vi "Ctr sys net adapter port auto detect.vi"(11 "HW Config IN":T1={"Dev. PC"=FALSE, "Swap XY on stage"=FALSE, "No of AOD"=0, "MC Supported"=FALSE, "Axial MC"=FALSE, "Computer MAC address"="", "Externalise Triggers"=FALSE, "Trigger HW config"={"Available Device List"=0, "Device Address"=""}, "DAQmx Chan"={"Pockels AO"="", "Hard shutter AO"="", "PMT AOs"="", "Galvo AOs"="", "Power meter AI"=""}, "XYZ Stage Control Config"=enum."None", "XY stage available"=FALSE, "XY Comms Config Cluster"={"Name"="COM7", "Device Address"="", "Port "=0, "Baudrate"=0, "Comms Type"=enum."GPIB-IEEE488"}, "Y stage available"=FALSE, "Y Comms Config Cluster"={"Name"="", "Device Address"="", "Port "=0, "Baudrate"=0, "Comms Type"=enum."GPIB-IEEE488"}, "Z stage available"=FALSE, "Z Comms Config Cluster "={"Name"="", "Device Address"="", "Port "=0, "Baudrate"=0, "Comms Type"=enum."GPIB-IEEE488"}, "Encoder available"=FALSE, "Encoder"={"IP address"="224.0.1.103", "Port"=7000, "Wheel radius (cm)"=16.0, "Encoder Trigger"=""}, "VidRec available"=FALSE, "Cam VidRec"={"DO flag-Video record"="", "DO flag-Trial start"=""}, "Laser Power Control HW config"={"Laser Power Control"="", "Laser Power Modulation Control"=enum."NI"}, "Laser 1 available"=FALSE, "Laser 1 config cluster"={"COM port"="COM7", "Baud Rate"=0, "Type"=""}, "Prechirper 1 available"=FALSE, "Prechirper 1 config cluster"={"Type"="", "Baud Rate"=0, "COM port"="COM7"}, "Control system.FPGA available?"=FALSE, "Control Sys. HW config"={"Control system.FPGA Type"=enum."Virtex 5", "Control system.Network adapter name"="", "Control system.MAC address"="", "Control system.Ethernet Port"=0, "Control system.Ethernet Port Opened"=FALSE}, "DAQ FPGA HW Config"={"FGPA Ref"=refnum, "Target"="RIO0", "input card type"=enum."AC Card"}, "PMT Control Voltage Limits"={"Lower Limit"=0.0, "Upper Limit"=0.0}} {"Encoder"."Wheel radius (cm)" format="%#_13g"}) -> (0 "error out":errorcluster, 3 "HW config OUT":T1={"Dev. PC"=FALSE, "Swap XY on stage"=FALSE, "No of AOD"=0, "MC Supported"=FALSE, "Axial MC"=FALSE, "Computer MAC address"="", "Externalise Triggers"=FALSE, "Trigger HW config"={"Available Device List"=0, "Device Address"=""}, "DAQmx Chan"={"Pockels AO"="", "Hard shutter AO"="", "PMT AOs"="", "Galvo AOs"="", "Power meter AI"=""}, "XYZ Stage Control Config"=enum."None", "XY stage available"=FALSE, "XY Comms Config Cluster"={"Name"="COM7", "Device Address"="", "Port "=0, "Baudrate"=0, "Comms Type"=enum."GPIB-IEEE488"}, "Y stage available"=FALSE, "Y Comms Config Cluster"={"Name"="", "Device Address"="", "Port "=0, "Baudrate"=0, "Comms Type"=enum."GPIB-IEEE488"}, "Z stage available"=FALSE, "Z Comms Config Cluster "={"Name"="", "Device Address"="", "Port "=0, "Baudrate"=0, "Comms Type"=enum."GPIB-IEEE488"}, "Encoder available"=FALSE, "Encoder"={"IP address"="224.0.1.103", "Port"=7000, "Wheel radius (cm)"=16.0, "Encoder Trigger"=""}, "VidRec available"=FALSE, "Cam VidRec"={"DO flag-Video record"="", "DO flag-Trial start"=""}, "Laser Power Control HW config"={"Laser Power Control"="", "Laser Power Modulation Control"=enum."NI"}, "Laser 1 available"=FALSE, "Laser 1 config cluster"={"COM port"="COM7", "Baud Rate"=0, "Type"=""}, "Prechirper 1 available"=FALSE, "Prechirper 1 config cluster"={"Type"="", "Baud Rate"=0, "COM port"="COM7"}, "Control system.FPGA available?"=FALSE, "Control Sys. HW config"={"Control system.FPGA Type"=enum."Virtex 5", "Control system.Network adapter name"="", "Control system.MAC address"="", "Control system.Ethernet Port"=0, "Control system.Ethernet Port Opened"=FALSE}, "DAQ FPGA HW Config"={"FGPA Ref"=refnum, "Target"="RIO0", "input card type"=enum."AC Card"}, "PMT Control Voltage Limits"={"Lower Limit"=0.0, "Upper Limit"=0.0}} {"Encoder"."Wheel radius (cm)" format="%#_13g"})   [LabVIEW 2020]
uses:
  Global Variables/General Globals.vi
  <vilib>/userDefined/High Color/nirio_resource_hc.ctl
  Typedefs/DAQmx physical channels cluster.ctl
  Typedefs/FPGA input type AC-DC.ctl
  Typedefs/Encoder config cluster.ctl
  Typedefs/Cam VidRec HW config setup cluster.ctl
  Typedefs/Control Sys HW config cluster.ctl
  Typedefs/Laser 1 config cluster.ctl
  Typedefs/PreChirper 1 config cluster.ctl
  Typedefs/Laser Power Control HW config.ctl
  Typedefs/Triggers HW config.ctl
  Typedefs/Hardware Configuration settings.ctl
  RIG-SPECIFIC FILES/FPGA Refs/FPGA Ref.ctl
  Typedefs/DAQ FPGA HW config cluster.ctl
  Typedefs/PMT Control Voltage limits.ctl
  Peripherals Control/XYZ Stage/Control/typedefs/XYZControlConfig.ctl
  Typedefs/Comms Type.ctl
  Typedefs/Peripherals comms config cluster.ctl
panel:
  out "Control system's network adapter name":string="82574L"
  out "Ethernet opened":bool
  out "# of enabled ports":i32
  out "Port Number":u32
  # "(make , model etc)"
  # "(COM Port / IP Address / service address etc.)"
  # "(Port for ethernet / channel for BT)"
  # "(make , model etc)"
  # "(COM Port / IP Address / service address etc.)"
  # "(Port for ethernet / channel for BT)"
  # "(make , model etc)"
  # "(COM Port / IP Address / service address etc.)"
  # "(Port for ethernet / channel for BT)"
  # "(make , model etc)"
  # "(COM Port / IP Address / service address etc.)"
  # "(Port for ethernet / channel for BT)"
  # "(make , model etc)"
  # "(COM Port / IP Address / service address etc.)"
  # "(Port for ethernet / channel for BT)"
  # "(make , model etc)"
  # "(COM Port / IP Address / service address etc.)"
  # "(Port for ethernet / channel for BT)"
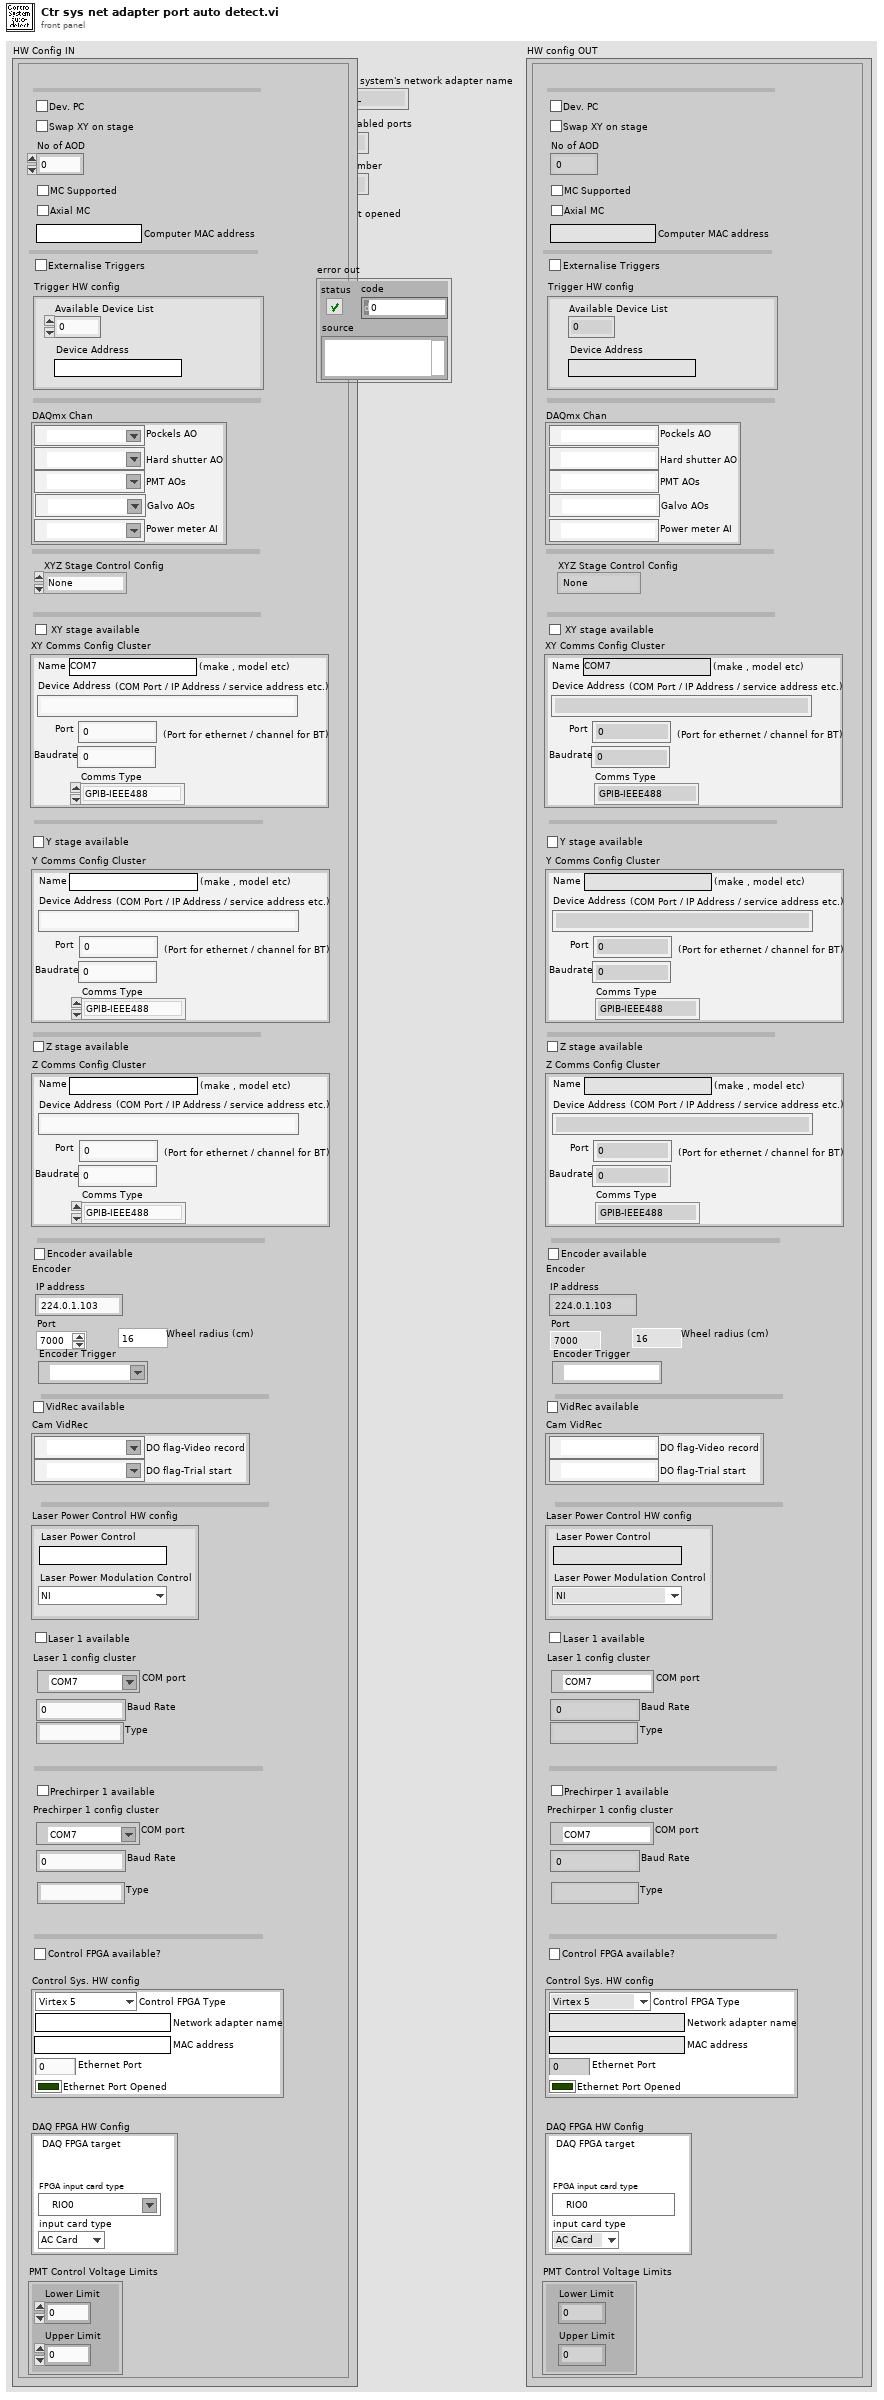
[diagram p1: front panel]
types:
  T1 = typedef "Hardware Configuration settings.ctl" = cluster{"Dev. PC":bool, "Swap XY on stage":bool, "No of AOD":u8, "MC Supported":bool, "Axial MC":bool, "Computer MAC address":string, "Externalise Triggers":bool, "Trigger HW config":T2, "DAQmx Chan":T3, "XYZ Stage Control Config":T4, "XY stage available":bool, "XY Comms Config Cluster":T5, "Y stage available":bool, "Y Comms Config Cluster":T5, "Z stage available":bool, "Z Comms Config Cluster ":T5, "Encoder available":bool, "Encoder":T7, "VidRec available":bool, "Cam VidRec":T8, "Laser Power Control HW config":T9, "Laser 1 available":bool, "Laser 1 config cluster":T10, "Prechirper 1 available":bool, "Prechirper 1 config cluster":T11, "Control system.FPGA available?":bool, "Control Sys. HW config":T12, "DAQ FPGA HW Config":T13, "PMT Control Voltage Limits":T17}
  T2 = typedef "Triggers HW config.ctl" = cluster{"Available Device List":i32, "Device Address":string}
  T3 = typedef "DAQmx physical channels cluster.ctl" = cluster{"Pockels AO":tag, "Hard shutter AO":tag, "PMT AOs":tag, "Galvo AOs":tag, "Power meter AI":tag}
  T4 = typedef "XYZControlConfig.ctl" = enum16{"None", "XYZ", "XY-Z", "X-Y-Z", "Z"}
  T5 = typedef "Peripherals comms config cluster.ctl" = cluster{"Name":string, "Device Address":string, "Port ":u16, "Baudrate":i32, "Comms Type":T6}
  T6 = typedef "Comms Type.ctl" = enum16{"GPIB-IEEE488", "Serial-RS232", "Serial-RS485", "Serial-RS422", "Serial-USB", "Ethernet-TCP/IP", "Ethernet-UDP"}
  T7 = typedef "Encoder config cluster.ctl" = cluster{"IP address":string, "Port":u16, "Wheel radius (cm)":dbl, "Encoder Trigger":tag}
  T8 = typedef "Cam VidRec HW config setup cluster.ctl" = cluster{"DO flag-Video record":tag, "DO flag-Trial start":tag}
  T9 = typedef "Laser Power Control HW config.ctl" = cluster{"Laser Power Control":string, "Laser Power Modulation Control":enum16{"NI", "FPGA"}}
  T10 = typedef "Laser 1 config cluster.ctl" = cluster{"COM port":refnum<visa-resource-name>, "Baud Rate":i32, "Type":string}
  T11 = typedef "PreChirper 1 config cluster.ctl" = cluster{"Type":string, "Baud Rate":i32, "COM port":refnum<visa-resource-name>}
  T12 = typedef "Control Sys HW config cluster.ctl" = cluster{"Control system.FPGA Type":enum16{"Virtex 5", "Virtex 7"}, "Control system.Network adapter name":string, "Control system.MAC address":string, "Control system.Ethernet Port":u32, "Control system.Ethernet Port Opened":bool}
  T13 = typedef "DAQ FPGA HW config cluster.ctl" = cluster{"FGPA Ref":T14, "Target":T15, "input card type":T16}
  T14 = typedef "FPGA Ref.ctl" = refnum<k20>
  T15 = typedef "nirio_resource_hc.ctl" = tag
  T16 = typedef "FPGA input type AC-DC.ctl" = enum16{"AC Card", "DC Card"}
  T17 = typedef "PMT Control Voltage limits.ctl" = cluster{"Lower Limit":dbl, "Upper Limit":dbl}
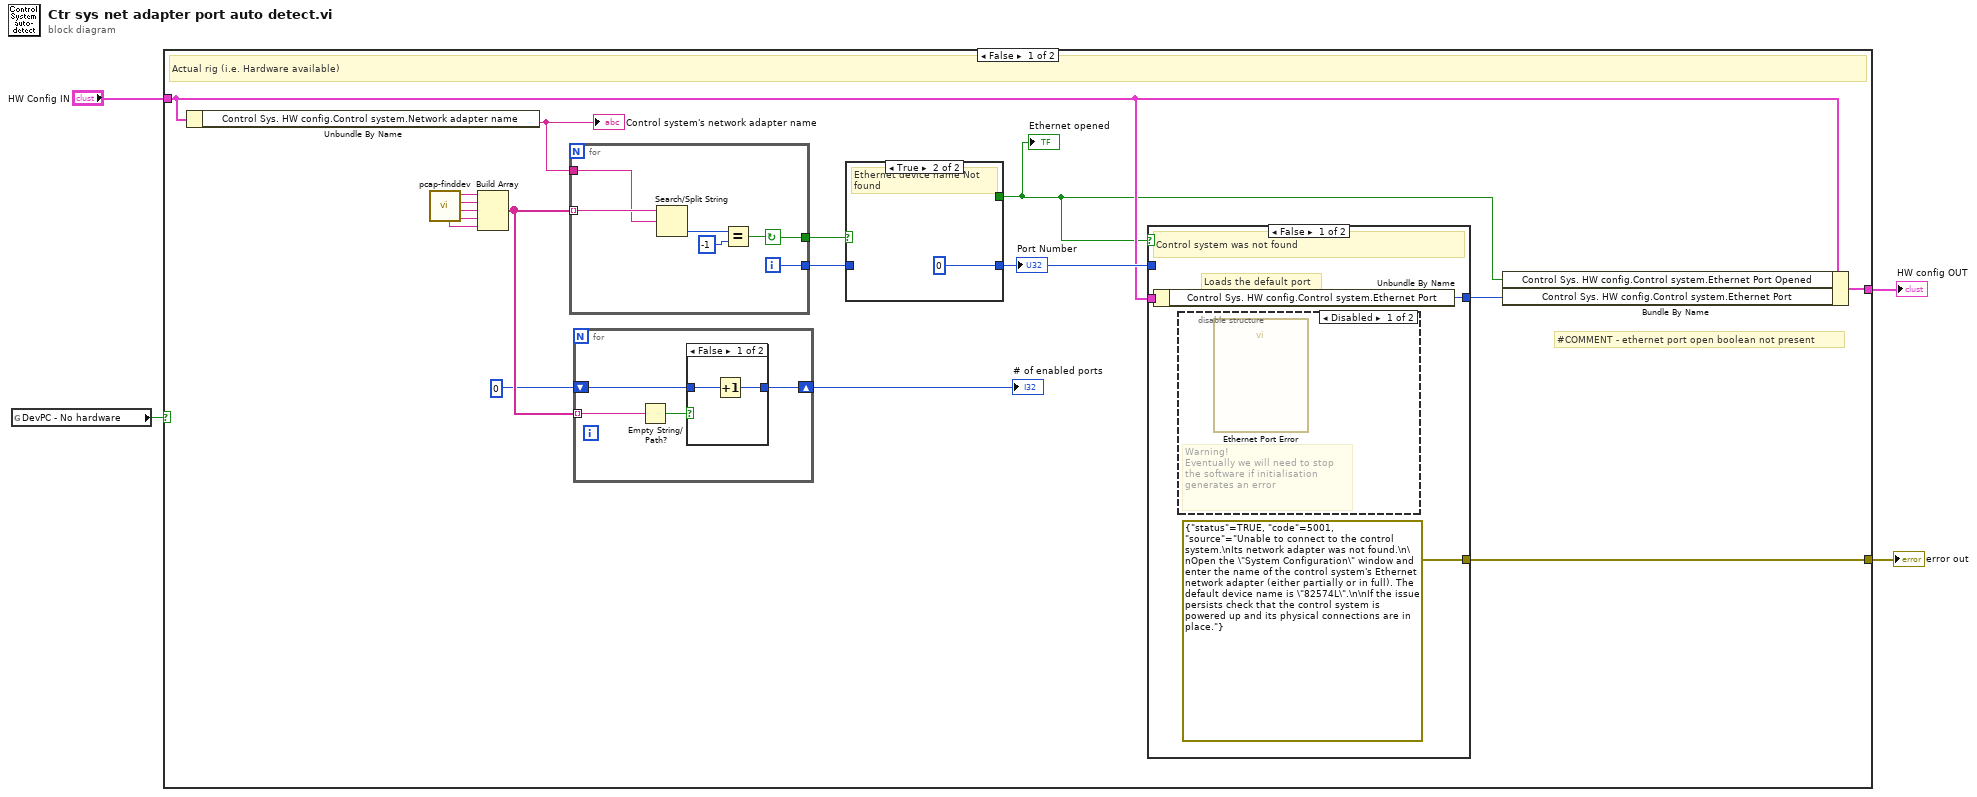
[diagram p0: block diagram]
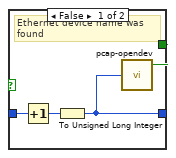
[diagram p5: hidden frame]
diagram:
  n1 = global read "General Globals.vi" "DevPC - No hardware"() -> (w2:bool)
  n2 = case shown="False" w2 {
    tunnel: [w11 w44] -> w1
    tunnel: "HW Config IN" -> [w9 w44]
    tunnel: [w8 _] -> w3
    frame False {
      # "#COMMENT - ethernet port open boolean not present"
      # "Actual rig (i.e. Hardware available)"
      n3 = Unbundle By Name(w9) -> ("Control Sys. HW config.Control system.Network adapter name"=w7:string)
      "Control system's network adapter name" <- w7
      n4 = call "pcap-finddev.vi"() -> ("String 4"=w18:string, "String 3"=w19:string, "String 2"=w20:string, "String"=w21:string, "String 5"=w17:string)  [unwired: 1 in]
      n5 = Build Array(w21, w20, w19, w18, w17) -> (w14:string[])
      n6 = for {
        tunnel: w14 -> [w39] mode=indexing
        tunnel: [w41] -> w16
        tunnel: [w40] -> w15
        tunnel: w7 -> [w38]
        i -> [w40]
        stop <- w41 continue-if-true
        n7 = Search/Split String(string=w39, search string/char (-)=w38) -> (offset of match=w43:i32)  [unwired: 1 in, 2 out]
        n8 = Equal?(x=w43, y=-1) -> (x = y?=w41:bool)
      }
      n9 = for {
        shift-right: [w28] -> w12
        shift-left: 0 -> [w27]
        tunnel: w14 -> [w26] mode=indexing
        n10 = Empty String/Path?(string/path=w26) -> (empty?=w29:bool)
        n11 = case shown="False" w29 {
          tunnel: [w31 w32] -> w28
          tunnel: w27 -> [w30 w32]
          frame False {
            n12 = Increment(x=w30) -> (x+1=w31:i32)
          }
          frame True {
          }
        }
      }
      "# of enabled ports" <- w12
      n13 = case shown="True" w16 {
        tunnel: w15 -> [w36 _]
        tunnel: [w33 u32 0] -> w10
        tunnel: [w35 _] -> w5
        frame False {
          # "Ethernet device name was found"
          n14 = Increment(x=w36) -> (x+1=w34:i32)
          n15 = To Unsigned Long Integer(number=w34) -> (unsigned 32bit integer=w33:u32)
          n16 = call "pcap-opendev.vi"("Select Device"=w33) -> ("Opened"=w35:bool)  [unwired: 2 out]
        }
        frame True {
          # "Ethernet device name Not found"
        }
      }
      "Port Number" <- w10
      "Ethernet opened" <- w5
      n17 = case shown="False" w5 {
        tunnel: [w23 w25] -> w6
        tunnel: w10 -> [_ w25]
        tunnel: w9 -> [w24 _]
        tunnel: [errorcluster {"status"=TRUE, "code"=5001, "source"="Unable to connect to the control system.\nIts network adapter was not found.\n\nOpen the \"System Configuration\" window and enter the name of the control system's Ethernet network adapter (either partially or in full). The default device name is \"82574L\".\n\nIf the issue persists check that the control system is powered up and its physical connections are in place."} ("error in (no error)") _] -> w8
        frame False {
          # "Loads the default port"
          # "Control system was not found"
          n18 = Unbundle By Name(w24) -> ("Control Sys. HW config.Control system.Ethernet Port"=w23:u32)
          n19 = disable-structure shown="Disabled" {
            frame Disabled {
              # "Warning!\nEventually we will need to stop the software if initialisation generates an error"
              n20 = call "Ethernet Port Error"() -> ()  [unwired: 18 in, 2 out]
            }
            frame Enabled {
            }
          }
        }
        frame True {
          # "Control system was found"
        }
      }
      n21 = Bundle By Name(cluster=w9, "Control Sys. HW config.Control system.Ethernet Port Opened"=w5, "Control Sys. HW config.Control system.Ethernet Port"=w6) -> (w11:T1)
    }
    frame True {
      # "Development Computer (i.e. No hardware available)"
    }
  }
  "error out" <- w3
  "HW config OUT" <- w1
